vi "Auto_Routine_Cube_Backup_Cube.vi"(8 "error in (no error)":errorcluster) -> (0 "error out":errorcluster)   [LabVIEW 2023]
uses:
  Arm/ArmPositionPreset.ctl
  Arm/ArmGamePiecePreset.ctl
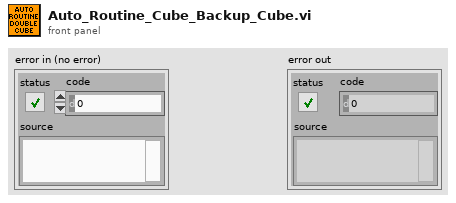
[diagram p1: front panel]
types:
  T1 = typedef "ArmGamePiecePreset.ctl" = enum16{"Cube", "Cone"}
  T2 = typedef "ArmPositionPreset.ctl" = enum16{"Upper", "Lower", "Middle", "Home", "Shelf", "Floor", "HalfFloor", "HalfHome"}
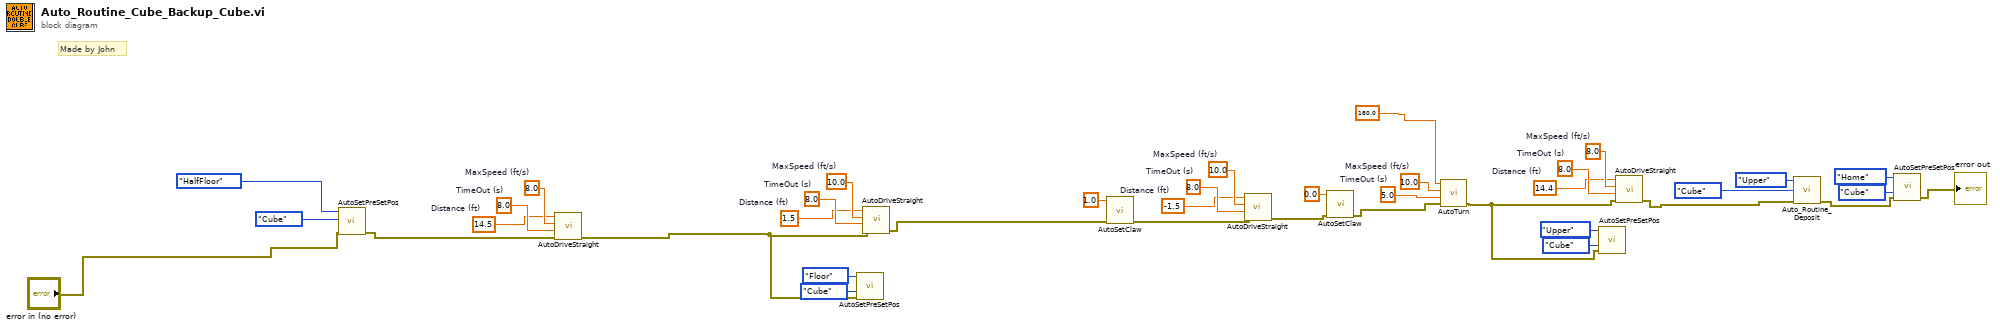
[diagram p0: block diagram]
diagram:
  w4 = 8.0  # TimeOut (s)
  w5 = 8.0  # MaxSpeed (ft/s)
  w3 = 14.4  # Distance (ft)
  w20 = 5.0  # TimeOut (s)
  w21 = 10.0  # MaxSpeed (ft/s)
  w25 = 8.0  # TimeOut (s)
  w26 = 10.0  # MaxSpeed (ft/s)
  w24 = -1.5  # Distance (ft)
  w28 = 8.0  # TimeOut (s)
  w29 = 10.0  # MaxSpeed (ft/s)
  w27 = 1.5  # Distance (ft)
  w37 = 8.0  # TimeOut (s)
  w38 = 8.0  # MaxSpeed (ft/s)
  w36 = 14.5  # Distance (ft)
  # "Made by John"
  n1 = call "AutoSetPreSetPos.vi"("error in (no error)"="error in (no error)", "Game Piece"=ArmGamePiecePreset."Cube", "Position"=ArmPositionPreset."HalfFloor") -> ("error out"=w6:errorcluster)  [unwired: 8 in]
  n2 = call "AutoDriveStraight.vi"("error in (no error)"=w6, "TimeOut (s)"=w37, "MaxSpeed (ft/s)"=w38, "Dist (ft)"=w36) -> ("error out"=w9:errorcluster)  [unwired: 7 in]
  n3 = call "AutoSetPreSetPos.vi"("error in (no error)"=w9, "Game Piece"=ArmGamePiecePreset."Cube", "Position"=ArmPositionPreset."Floor") -> ()  [unwired: 8 in, 1 out]
  n4 = call "AutoDriveStraight.vi"("error in (no error)"=w9, "TimeOut (s)"=w28, "MaxSpeed (ft/s)"=w29, "Dist (ft)"=w27) -> ("error out"=w10:errorcluster)  [unwired: 7 in]
  n5 = call "AutoSetClaw.vi"("error in (no error)"=w10, "ClawDemand"=1.0) -> ("error out"=w23:errorcluster)  [unwired: 9 in]
  n6 = call "AutoDriveStraight.vi"("error in (no error)"=w23, "TimeOut (s)"=w25, "MaxSpeed (ft/s)"=w26, "Dist (ft)"=w24) -> ("error out"=w22:errorcluster)  [unwired: 7 in]
  n7 = call "AutoSetClaw.vi"("error in (no error)"=w22, "ClawDemand"=0.0) -> ("error out"=w11:errorcluster)  [unwired: 9 in]
  n8 = call "AutoTurn.vi"("error in (no error)"=w11, "TimeOut (s)"=w20, "MaxSpeed (ft/s)"=w21, "degrees"=180.0) -> ("error out"=w1:errorcluster)  [unwired: 7 in]
  n9 = call "AutoSetPreSetPos.vi"("error in (no error)"=w1, "Game Piece"=ArmGamePiecePreset."Cube", "Position"=ArmPositionPreset."Upper") -> ()  [unwired: 8 in, 1 out]
  n10 = call "AutoDriveStraight.vi"("error in (no error)"=w1, "TimeOut (s)"=w4, "MaxSpeed (ft/s)"=w5, "Dist (ft)"=w3) -> ("error out"=w2:errorcluster)  [unwired: 7 in]
  n11 = call "Auto_Routine_Deposit.vi"("error in (no error)"=w2, "Game Piece"=ArmGamePiecePreset."Cube", "Position"=ArmPositionPreset."Upper") -> ("error out"=w15:errorcluster)  [unwired: 8 in]
  n12 = call "AutoSetPreSetPos.vi"("error in (no error)"=w15, "Game Piece"=ArmGamePiecePreset."Cube", "Position"=ArmPositionPreset."Home") -> ("error out"=→"error out":errorcluster)  [unwired: 8 in]
